vi "Export Image.vi"(0 "Display State In":T1, 5 "File Type":enum32{"BMP", "EPS", "EMF", "PICT"}(ring), 7 "Target":enum32{"File", "Clipboard"}(ring), 9 "Container State":T3, 11 "error in (no error)":errorcluster, 12 "Path":path, 13 "Hide Grid":bool, 14 "Always Overwrite":bool) -> (4 "Display State Out":T1, 15 "error out":errorcluster)   [LabVIEW 2020, in "XY Plot Matrix.xctl"]
uses:
  <vilib>/Math Plots/2D Math Plots/XY Plot Matrix/XY Plot Matrix XCtrl/XY Plot Matrix.xctl
  <vilib>/_xctls/Container State.ctl
  <vilib>/Math Plots/2D Math Plots/XY Plot Matrix/XY Plot Matrix XCtrl/State.ctl
  <vilib>/Math Plots/2D Math Plots/XY Plot Matrix/XY Plot Matrix/XY Plot Matrix.lvclass
  <vilib>/Math Plots/2D Math Plots/2D Plot/Action String/XYPlotMatrix Ctrl Act Queue.ctl
  <vilib>/Math Plots/2D Math Plots/2D Plot/Action String/XYPlotMatrix Ctrl Act Cluster.ctl
  <vilib>/Math Plots/2D Math Plots/2D Plot/Action String/2DMathPlot State Class.ctl
  <vilib>/_xctls/XControlSupport.lvlib
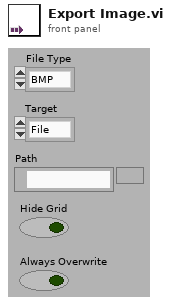
[diagram p1: front panel]
types:
  T1 = typedef "XY Plot Matrix.xctl/State.ctl" = cluster{"XY Plot Matrix.lvclass":refnum<class "XY Plot Matrix.lvclass">, "Control Ref Queue":T2, "Main Frame Color":u32}
  T2 = typedef "XYPlotMatrix Ctrl Act Queue.ctl" = refnum<queue>
  T3 = typedef "XControlSupport.lvlib/Container State.ctl" = cluster{"Indicator?":bool, "Run Mode?":bool, " Refnum":refnum<vi>}
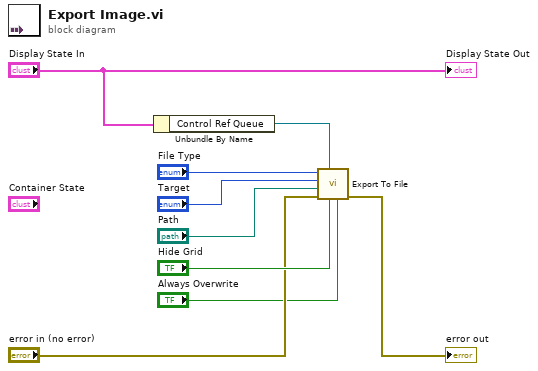
[diagram p0: block diagram]
diagram:
  n1 = Unbundle By Name("Display State In") -> ("Control Ref Queue"=w5:T2)
  n2 = call <vilib>:"Export To File.vi"("Always Overwrite"="Always Overwrite", "Hide Grid"="Hide Grid", "Control Ref Queue"=w5, "error in (no error)"="error in (no error)", "Path"="Path", "Target"="Target", "File Type"="File Type") -> ("error out"=→"error out":errorcluster)  [unwired: 4 out]
  "Display State Out" <- "Display State In"
